vi "Generic command handler.vi"(8 "error in (no error)":errorcluster, 10 "Message in":refnum<class "GenericMessage.lvclass">, 11 "Tomo in":refnum<class "Tomo.lvclass">) -> (0 "error out":errorcluster, 2 "value":string, 3 "Tomo out":refnum<class "Tomo.lvclass">)   [LabVIEW 2012, in "Tomo.lvclass"]
doc: "The generic_command_handler processes the command 'generic'. Commands which are not part of the predefined list of commands fall under the 'generic' command for special activity."
uses:
  Tomo.lvclass
  <vilib>/Distrio/Murmex/GenericMessage/GenericMessage.lvclass
  <vilib>/Distrio/Murmex/Murmex/Murmex.lvclass
  Tomo.lvclass/Tomo.ctl
  <vilib>/Distrio/Murmex/StartMessage/StartMessage.lvclass
  Current activity.ctl
  file type.ctl
  notice type.ctl
  <vilib>/Distrio/Murmex/StopMessage/StopMessage.lvclass
  <vilib>/Distrio/Murmex/Message/Add or replace parameter.vi
  <vilib>/Distrio/Murmex/Message/Message.lvclass
  <vilib>/vision/NI_Vision_Development_Module.lvlib
panel:
  out "Image 2":T1(plugin-control)
  out "Image":T1(plugin-control)
  # "This method is called when the GENERIC\ntrigger is sent. \n\nOverride this method when your component needs to\nrespond to this trigger. \n\nCall parent for proper implementation"
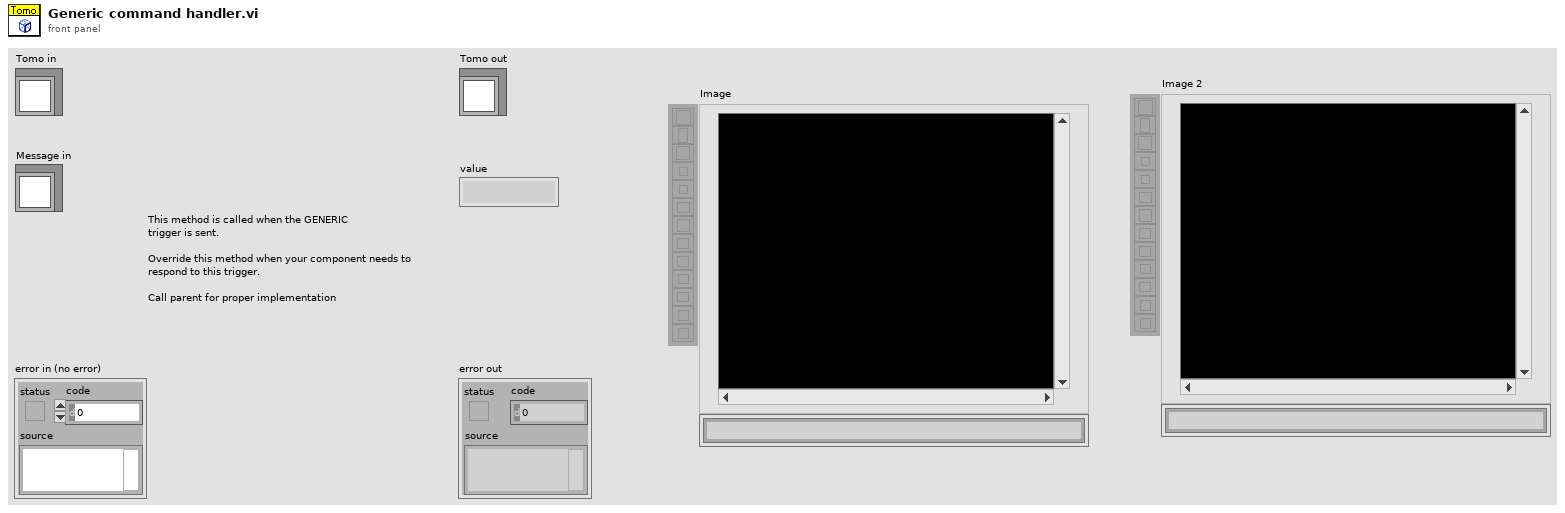
[diagram p1: front panel]
types:
  T1 = typedef "IMAQ Image.ctl" = refnum<image>
  T2 = typedef "Tomo.lvclass/Current activity.ctl" = enum16{"Idle", "Inter-stack motion", "Pre-tomo calculation", "Stack acquisition", "Stack preparation", "Pre-tomo stack acq", "Pre-tomo inter-stack"}
  T3 = typedef "Tomo.lvclass/file type.ctl" = enum16{"Volume map", "Completed stacks"}
  T4 = typedef "Tomo.lvclass/notice type.ctl" = enum16{"Tomography stopped", "Tomography error", "Tomography finished", "Timing issue", "Critical timing issue"}
  T5 = typedef "Tomo.lvclass/volume map.ctl" = enum16{"Cubic volume", "Custom volume", "Self-generate volume"}
  T6 = cluster{"Mean Value":sgl, "Standard Variation":sgl, "Minimal Value":sgl, "Maximal Value":sgl, "Area (calibrated)":sgl, "Area (pixels)":u32, "%":sgl, "Calibration Valid":bool}
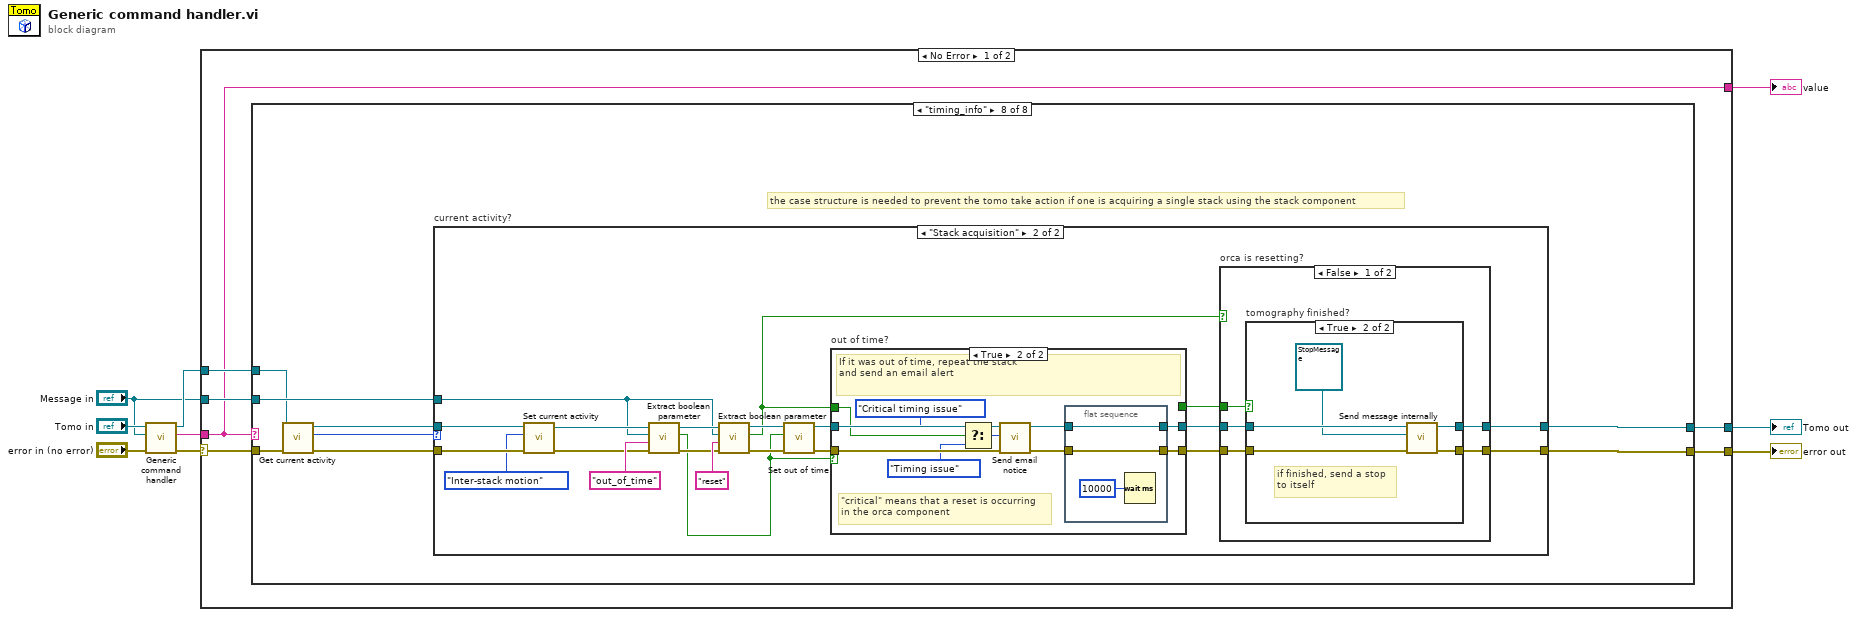
[diagram p0: block diagram]
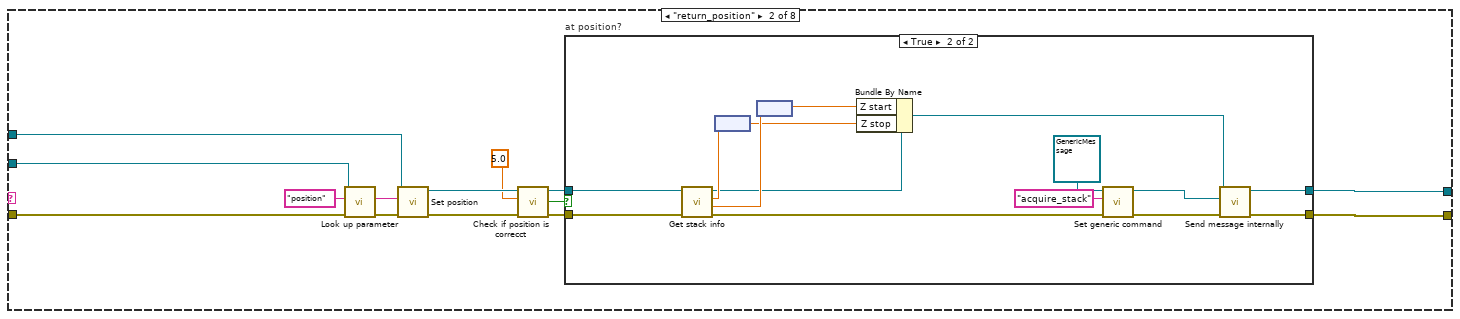
[diagram p3: hidden frame]
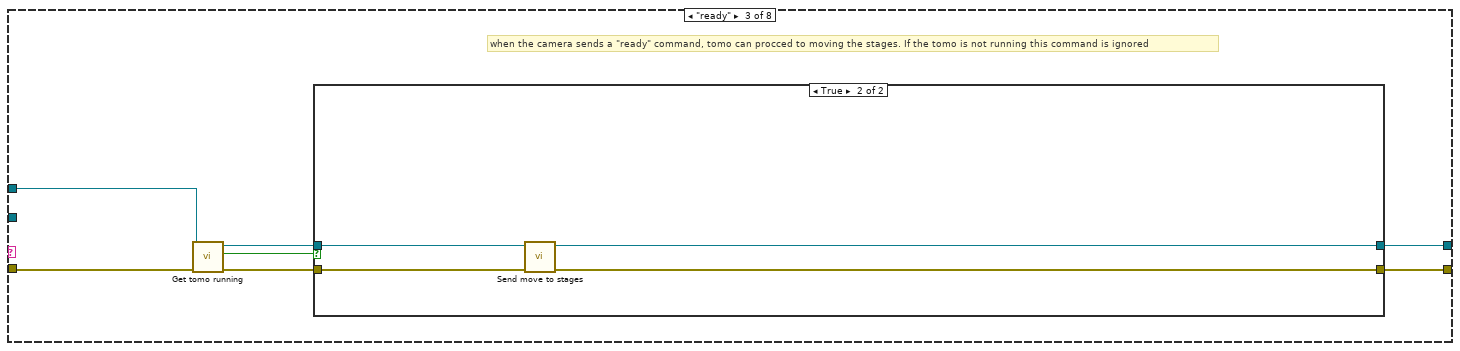
[diagram p5: hidden frame]
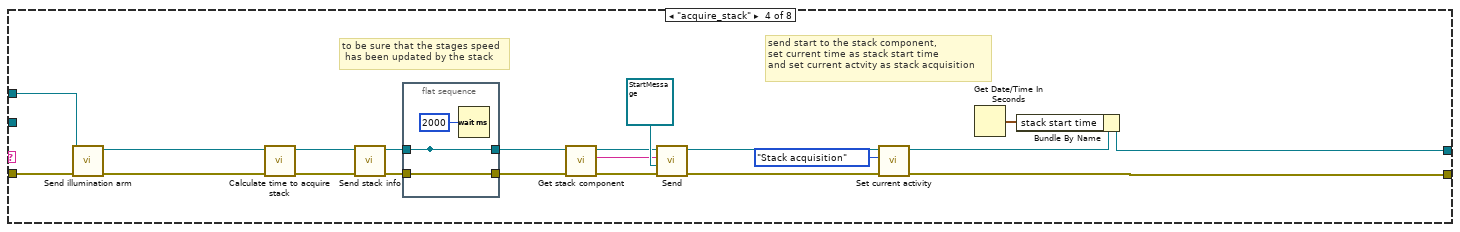
[diagram p7: hidden frame]
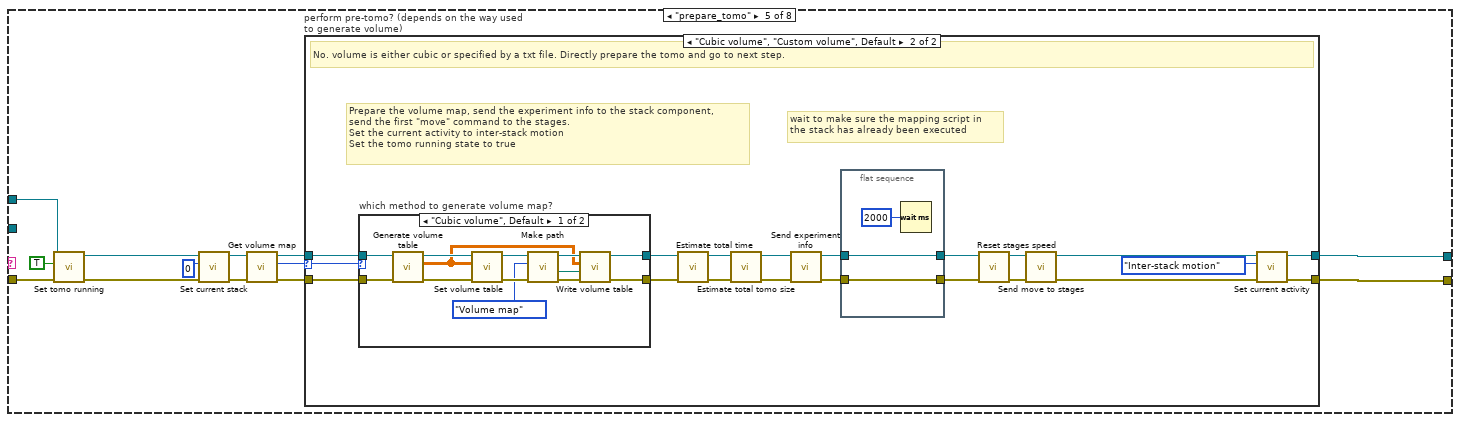
[diagram p8: hidden frame]
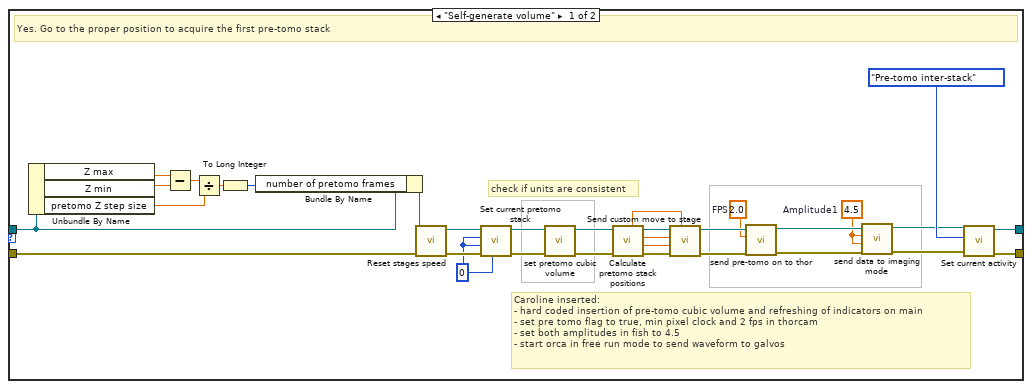
[diagram p9: hidden frame]
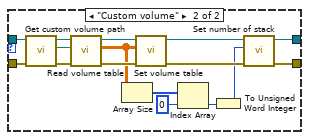
[diagram p10: hidden frame]
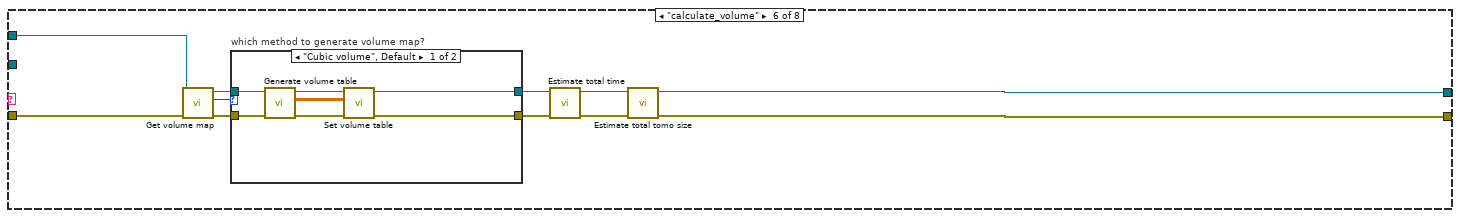
[diagram p11: hidden frame]
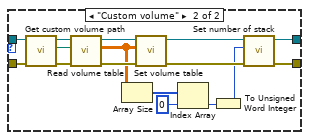
[diagram p12: hidden frame]
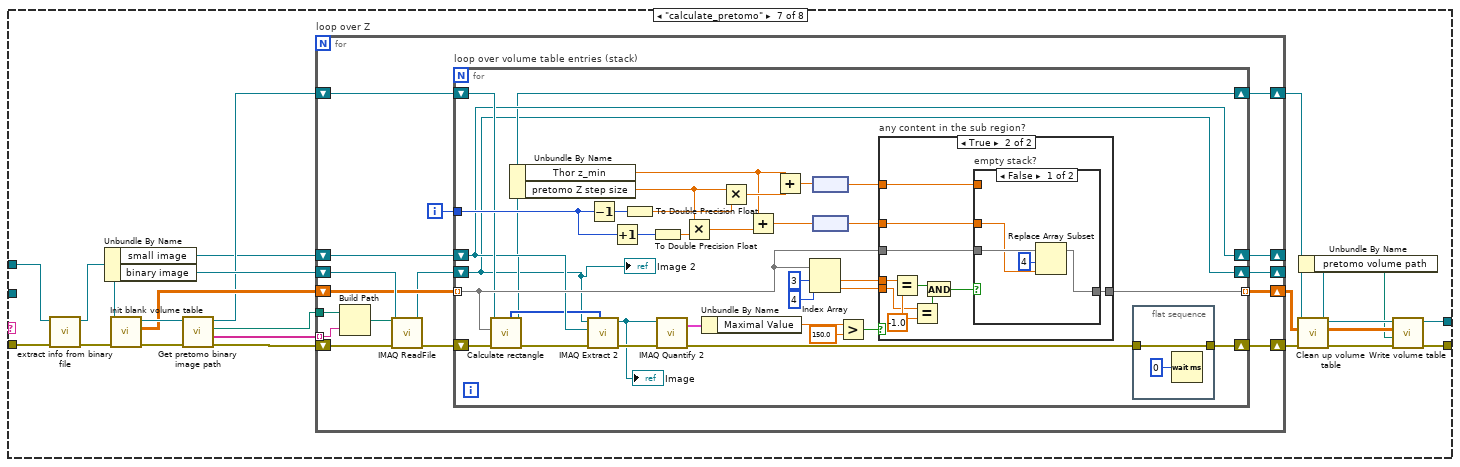
[diagram p13: hidden frame]
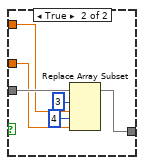
[diagram p15: hidden frame]
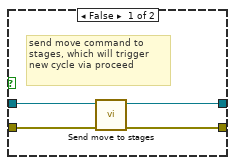
[diagram p17: hidden frame]
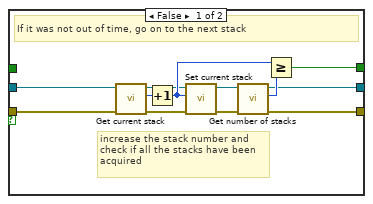
[diagram p19: hidden frame]
diagram:
  n1 = call-parent "Generic command handler.vi"("error in (no error)"="error in (no error)", "Message in"="Message in", "Murmex in"="Tomo in") -> ("error out"=w7:errorcluster, "value"=w6:string, "Murmex out"=w5:refnum<class "Tomo.lvclass">)  [unwired: 6 in]
  n2 = case shown="No Error" w7 {
    selector: w7 -> [w15 w384]
    tunnel: w6 -> [w11 w386]
    tunnel: w5 -> [w14 w385]
    tunnel: "Message in" -> [w13 _]
    tunnel: [w12 w385] -> w3
    tunnel: [w11 w386] -> w2
    tunnel: [w10 w384] -> w1
    frame No Error {
      n3 = case shown="\"timing_info\"" w11 {
        tunnel: w15 -> [w17 w31 w55 w66 w89 w186 w223 w316]
        tunnel: w14 -> [w16 w30 w54 w68 w90 w185 w221 w314]
        tunnel: w13 -> [_ w29 _ _ _ _ _ w319]
        tunnel: [w17 w19 w51 w79 w88 w183 w227 w317] -> w10
        tunnel: [w16 w18 w49 w62 w87 w184 w229 w318] -> w12
        frame Default {
        }
        frame "return_position" {
          n4 = call <vilib>:"Look up parameter.vi"("error in (no error)"=w31, "name"="position", "Message in"=w29) -> ("error out"=w27:errorcluster, "key"=w26:string)  [unwired: 5 in, 2 out]
          n5 = call-dynamic "Set position.vi"("error in (no error)"=w27, "XML in"=w26, "Tomo in"=w30) -> ("error out"=w25:errorcluster, "Tomo out"=w24:refnum<class "Tomo.lvclass">)  [unwired: 7 in]
          n6 = call-dynamic "Check if position is correcct.vi"("error in (no error)"=w25, "Tolerance (um)"=5.0 ("Tolerance"), "Tomo in"=w24) -> ("error out"=w21:errorcluster, "correct?"=w22:bool, "Tomo out"=w20:refnum<class "Tomo.lvclass">)  [unwired: 6 in]
          n7 = case "at position?" shown="True" w22 {
            tunnel: w21 -> [w33 w34]
            tunnel: w20 -> [w32 w35]
            tunnel: [w33 w48] -> w19
            tunnel: [w32 w47] -> w18
            frame False {
            }
            frame True {
              n8 = call-dynamic "Get stack info.vi"("error in (no error)"=w34, "Tomo in"=w35) -> ("error out"=w38:errorcluster, "Z start"=w45:dbl, "Z stop"=w46:dbl, "Tomo out"=w36:refnum<class "Tomo.lvclass">)  [unwired: 4 in, 2 out]
              n9 = node(w46) -> (w43:dbl[unit])
              n10 = node(w45) -> (w44:dbl[unit])
              n11 = Bundle By Name(cluster=w36, "Z start"=w44, "Z stop"=w43) -> (w37:refnum<class "Tomo.lvclass">)
              n12 = call <vilib>:"Set generic command.vi"("error in (no error)"=w38, "generic command"="acquire_stack", "GenericMessage in"=refnum<class "GenericMessage.lvclass"> refnum ("Distrio Murmex 1.2:GenericMessage")) -> ("error out"=w42:errorcluster, "GenericMessage out"=w39:refnum<class "GenericMessage.lvclass">)  [unwired: 7 in]
              n13 = call <vilib>:"Send message internally.vi"("error in (no error)"=w42, "Message"=w39, "Murmex in"=w37) -> ("error out"=w48:errorcluster, "Murmex out"=w47:refnum<class "Tomo.lvclass">)  [unwired: 7 in]
            }
          }
        }
        frame "ready" {
          # "when the camera sends a \"ready\" command, tomo can procced to moving the stages. If the tomo is not running this command is ignored"
          n14 = call-dynamic "Get tomo running.vi"("error in (no error)"=w55, "Tomo in"=w54) -> ("error out"=w52:errorcluster, "tomo running?"=w53:bool, "Tomo out"=w50:refnum<class "Tomo.lvclass">)  [unwired: 7 in]
          n15 = case shown="True" w53 {
            tunnel: w52 -> [w56 w61]
            tunnel: [w56 w60] -> w51
            tunnel: w50 -> [w57 w59]
            tunnel: [w57 w58] -> w49
            frame False {
            }
            frame True {
              n16 = call-dynamic "Send move to stages.vi"("error in (no error)"=w61, "Tomo in"=w59) -> ("error out"=w60:errorcluster, "Tomo out"=w58:refnum<class "Tomo.lvclass">)  [unwired: 8 in]
            }
          }
        }
        frame "acquire_stack" {
          # "to be sure that the stages speed\n has been updated by the stack"
          # "send start to the stack component,\nset current time as stack start time\nand set current actvity as stack acquisition"
          n17 = call-dynamic "Send illumination arm.vi"("error in (no error)"=w66, "Tomo in"=w68) -> ("error out"=w74:errorcluster, "Tomo out"=w73:refnum<class "Tomo.lvclass">)  [unwired: 8 in]
          n18 = call-dynamic "Calculate time to acquire stack.vi"("error in (no error)"=w74, "Tomo in"=w73) -> ("error out"=w65:errorcluster, "Tomo out"=w69:refnum<class "Tomo.lvclass">)  [unwired: 8 in]
          n19 = call-dynamic "Send stack info.vi"("error in (no error)"=w65, "Tomo in"=w69) -> ("error out"=w72:errorcluster, "Tomo out"=w71:refnum<class "Tomo.lvclass">)  [unwired: 8 in]
          n20 = flat-sequence {
            tunnel: [w85] -> w64
            tunnel: w72 -> [w85]
            tunnel: w71 -> [w83]
            tunnel: [w83] -> _
            tunnel: [w83] -> w67
            frame #0 {
              n21 = Wait (ms)(milliseconds to wait=u32 2000) -> ()  [unwired: 1 out]
            }
          }
          n22 = call-dynamic "Get stack component.vi"("error in (no error)"=w64, "Tomo in"=w67) -> ("error out"=w75:errorcluster, "stack component"=w81:string, "Tomo out"=w76:refnum<class "Tomo.lvclass">)  [unwired: 7 in]
          n23 = call <vilib>:"Send.vi"("error in (no error)"=w75, "Message"=refnum<class "StartMessage.lvclass"> refnum ("Message in"), "recipient"=w81, "Murmex in"=w76) -> ("error out"=w80:errorcluster, "Murmex out"=w78:refnum<class "Tomo.lvclass">)  [unwired: 6 in]
          n24 = call-dynamic "Set current activity.vi"("error in (no error)"=w80, "Current activity"=Current_activity."Stack acquisition", "Tomo in"=w78) -> ("error out"=w79:errorcluster, "Tomo out"=w63:refnum<class "Tomo.lvclass">)  [unwired: 7 in]
          n25 = Get Date/Time In Seconds() -> (seconds since 1Jan1904=w70:timestamp)
          n26 = Bundle By Name(cluster=w63, "stack start time"=w70) -> (w62:refnum<class "Tomo.lvclass">)
        }
        frame "prepare_tomo" {
          n27 = call-dynamic "Set tomo running.vi"("error in (no error)"=w89, "tomo running?"=TRUE, "Tomo in"=w90) -> ("error out"=w91:errorcluster, "Tomo out"=w92:refnum<class "Tomo.lvclass">)  [unwired: 7 in]
          n28 = call-dynamic "Set current stack.vi"("error in (no error)"=w91, "Current stack"=u16 0, "Tomo in"=w92) -> ("error out"=w95:errorcluster, "Tomo out"=w96:refnum<class "Tomo.lvclass">)  [unwired: 7 in]
          n29 = call-dynamic "Get volume map.vi"("error in (no error)"=w95, "Tomo in"=w96) -> ("error out"=w98:errorcluster, "Volume map"=w86:T5, "Tomo out"=w97:refnum<class "Tomo.lvclass">)  [unwired: 7 in]
          n30 = case "perform pre-tomo? (depends on the way used to generate volume)" shown="\"Cubic volume\", \"Custom volume\", Default" w86 {
            selector: w86 -> [_ w131]
            tunnel: w98 -> [w111 w150]
            tunnel: w97 -> [w112 w149]
            tunnel: [w123 w141] -> w88
            tunnel: [w122 w139] -> w87
            frame "Self-generate volume" {
              w105 = 2.0  # FPS
              w106 = 4.5  # Amplitude1
              w113 = 0 ("current x stack")
              # "Caroline inserted:\n- hard coded insertion of pre-tomo cubic volume and refreshing of indicators on main\n- set pre tomo flag to true, min pixel clock and 2 fps in thorcam\n- set both amplitudes in fish to 4.5\n- start orca in free run mode to send waveform to galvos"
              # "check if units are consistent"
              # "Yes. Go to the proper position to acquire the first pre-tomo stack"
              n31 = Unbundle By Name(w112) -> ("Z max"=w120:dbl[unit], "Z min"=w119:dbl[unit], "pretomo Z step size"=w117:dbl[unit])
              n32 = Subtract(x=w120, y=w119) -> (x-y=w118:dbl[unit])
              n33 = Divide(x=w118, y=w117) -> (x/y=w114:dbl)
              n34 = To Long Integer(number=w114) -> (32bit integer=w115:i32)
              n35 = Bundle By Name(cluster=w112, "number of pretomo frames"=w115) -> (w116:refnum<class "Tomo.lvclass">)
              n36 = call-dynamic "Reset stages speed.vi"("error in (no error)"=w111, "Tomo in"=w116) -> ("error out"=w130:errorcluster, "Tomo out"=w129:refnum<class "Tomo.lvclass">)  [unwired: 8 in]
              n37 = call-dynamic "Set current pretomo stack.vi"("z step number"=w113, "error in (no error)"=w130, "current y stack"=w113, "current x stack"=w113, "Tomo in"=w129) -> ("error out"=w102:errorcluster, "Tomo out"=w104:refnum<class "Tomo.lvclass">)  [unwired: 5 in]
              n38 = call-dynamic "set pretomo cubic volume.vi"("error in (no error)"=w102, "Tomo in"=w104) -> ("error out"=w101:errorcluster, "Tomo out"=w103:refnum<class "Tomo.lvclass">)  [unwired: 8 in]
              n39 = call-dynamic "Calculate pretomo stack positions.vi"("error in (no error)"=w101, "Tomo in"=w103) -> ("error out"=w127:errorcluster, "Y pos"=w124:dbl[unit], "X pos"=w125:dbl[unit], "Tomo out"=w128:refnum<class "Tomo.lvclass">, "Z pos"=w126:dbl[unit])  [unwired: 5 in]
              n40 = call-dynamic "Send custom move to stage.vi"("Z pos"=w126, "error in (no error)"=w127, "Y pos"=w124, "X pos"=w125, "Tomo in"=w128) -> ("error out"=w110:errorcluster, "Tomo out"=w109:refnum<class "Tomo.lvclass">)  [unwired: 5 in]
              n41 = call-dynamic "send pre-tomo on to thor.vi"("error in (no error)"=w110, "FPS"=w105, "Tomo in"=w109) -> ("error out"=w107:errorcluster, "Tomo out"=w108:refnum<class "Tomo.lvclass">)  [unwired: 7 in]
              n42 = call-dynamic "send data to imaging mode.vi"("error in (no error)"=w107, "Amplitude2"=w106, "Amplitude1"=w106, "Tomo in"=w108) -> ("error out"=w100:errorcluster, "Tomo out"=w99:refnum<class "Tomo.lvclass">)  [unwired: 6 in]
              n43 = call-dynamic "Set current activity.vi"("error in (no error)"=w100, "Current activity"=Current_activity."Pre-tomo inter-stack", "Tomo in"=w99) -> ("error out"=w123:errorcluster, "Tomo out"=w122:refnum<class "Tomo.lvclass">)  [unwired: 7 in]
            }
            frame "Cubic volume", "Custom volume", Default {
              # "wait to make sure the mapping script in \nthe stack has already been executed"
              # "Prepare the volume map, send the experiment info to the stack component,\nsend the first \"move\" command to the stages.\nSet the current activity to inter-stack motion\nSet the tomo running state to true"
              # "No. volume is either cubic or specified by a txt file. Directly prepare the tomo and go to next step."
              n44 = case "which method to generate volume map?" shown="\"Cubic volume\", Default" w131 {
                tunnel: w150 -> [w165 w180]
                tunnel: w149 -> [w166 w178]
                tunnel: [w155 w172] -> w147
                tunnel: [w154 w174] -> w148
                frame "Cubic volume", Default {
                  n45 = call-dynamic "Generate volume table.vi"("error in (no error)"=w165, "Tomo in"=w166) -> ("error out"=w163:errorcluster, "Volume table"=w156:dbl[][], "Tomo out"=w164:refnum<class "Tomo.lvclass">)  [unwired: 7 in]
                  n46 = call-dynamic "Set volume table.vi"("error in (no error)"=w163, "Volume map in"=w156, "Tomo in"=w164) -> ("error out"=w161:errorcluster, "Tomo out"=w162:refnum<class "Tomo.lvclass">)  [unwired: 7 in]
                  n47 = call-dynamic "Make path.vi"("error in (no error)"=w161, "File type"=file_type."Volume map", "Tomo in"=w162) -> ("error out"=w158:errorcluster, "path"=w157:path, "Tomo out"=w159:refnum<class "Tomo.lvclass">)  [unwired: 6 in]
                  n48 = call-dynamic "Write volume table.vi"("error in (no error)"=w158, "File name"=w157, "Volume map"=w156, "Tomo in"=w159) -> ("error out"=w154:errorcluster, "Tomo out"=w155:refnum<class "Tomo.lvclass">)  [unwired: 6 in]
                }
                frame "Custom volume" {
                  n49 = call-dynamic "Get custom volume path.vi"("error in (no error)"=w180, "Tomo in"=w178) -> ("error out"=w179:errorcluster, "Custom volume path"=w176:path, "Tomo out"=w177:refnum<class "Tomo.lvclass">)  [unwired: 7 in]
                  n50 = call "Read volume table.vi"("error in (no error)"=w179, "File path"=w176, "Tomo in"=w177) -> ("error out"=w181:errorcluster, "System Array"=w168:dbl[][], "Tomo out"=w182:refnum<class "Tomo.lvclass">)  [unwired: 6 in]
                  n51 = Array Size(array=w168) -> (size(s)=w171:i32[])
                  n52 = call-dynamic "Set volume table.vi"("error in (no error)"=w181, "Volume map in"=w168, "Tomo in"=w182) -> ("error out"=w175:errorcluster, "Tomo out"=w173:refnum<class "Tomo.lvclass">)  [unwired: 7 in]
                  n53 = Index Array(array=w171, index=0) -> (element=w169:i32)
                  n54 = To Unsigned Word Integer(number=w169) -> (unsigned 16bit integer=w167:u16)
                  n55 = call-dynamic "Set number of stack.vi"("error in (no error)"=w175, "Number of stacks"=w167, "Tomo in"=w173) -> ("error out"=w174:errorcluster, "Tomo out"=w172:refnum<class "Tomo.lvclass">)  [unwired: 7 in]
                }
              }
              n56 = call-dynamic "Estimate total time.vi"("error in (no error)"=w148, "Tomo in"=w147) -> ("error out"=w135:errorcluster, "Tomo out"=w137:refnum<class "Tomo.lvclass">)  [unwired: 7 in, 1 out]
              n57 = call "Estimate total tomo size.vi"("error in (no error)"=w135, "Tomo in"=w137) -> ("error out"=w134:errorcluster, "Tomo out"=w136:refnum<class "Tomo.lvclass">)  [unwired: 7 in, 1 out]
              n58 = call-dynamic "Send experiment info.vi"("error in (no error)"=w134, "Tomo in"=w136) -> ("error out"=w142:errorcluster, "Tomo out"=w144:refnum<class "Tomo.lvclass">)  [unwired: 8 in]
              n59 = flat-sequence {
                tunnel: [w153] -> w145
                tunnel: w144 -> [w153]
                tunnel: [w152] -> w143
                tunnel: w142 -> [w152]
                frame #0 {
                  n60 = Wait (ms)(milliseconds to wait=u32 2000) -> ()  [unwired: 1 out]
                }
              }
              n61 = call-dynamic "Reset stages speed.vi"("error in (no error)"=w143, "Tomo in"=w145) -> ("error out"=w133:errorcluster, "Tomo out"=w132:refnum<class "Tomo.lvclass">)  [unwired: 8 in]
              n62 = call-dynamic "Send move to stages.vi"("error in (no error)"=w133, "Tomo in"=w132) -> ("error out"=w146:errorcluster, "Tomo out"=w140:refnum<class "Tomo.lvclass">)  [unwired: 8 in]
              n63 = call-dynamic "Set current activity.vi"("error in (no error)"=w146, "Current activity"=Current_activity."Inter-stack motion", "Tomo in"=w140) -> ("error out"=w141:errorcluster, "Tomo out"=w139:refnum<class "Tomo.lvclass">)  [unwired: 7 in]
            }
          }
        }
        frame "calculate_volume" {
          n64 = call-dynamic "Get volume map.vi"("error in (no error)"=w186, "Tomo in"=w185) -> ("error out"=w192:errorcluster, "Volume map"=w193:T5, "Tomo out"=w191:refnum<class "Tomo.lvclass">)  [unwired: 7 in]
          n65 = case "which method to generate volume map?" shown="\"Cubic volume\", Default" w193 {
            tunnel: w192 -> [w199 w214]
            tunnel: w191 -> [w200 w212]
            tunnel: [w195 w206] -> w189
            tunnel: [w194 w208] -> w190
            frame "Cubic volume", Default {
              n66 = call-dynamic "Generate volume table.vi"("error in (no error)"=w199, "Tomo in"=w200) -> ("error out"=w197:errorcluster, "Volume table"=w196:dbl[][], "Tomo out"=w198:refnum<class "Tomo.lvclass">)  [unwired: 7 in]
              n67 = call-dynamic "Set volume table.vi"("error in (no error)"=w197, "Volume map in"=w196, "Tomo in"=w198) -> ("error out"=w194:errorcluster, "Tomo out"=w195:refnum<class "Tomo.lvclass">)  [unwired: 7 in]
            }
            frame "Custom volume" {
              n68 = call-dynamic "Get custom volume path.vi"("error in (no error)"=w214, "Tomo in"=w212) -> ("error out"=w213:errorcluster, "Custom volume path"=w210:path, "Tomo out"=w211:refnum<class "Tomo.lvclass">)  [unwired: 7 in]
              n69 = call "Read volume table.vi"("error in (no error)"=w213, "File path"=w210, "Tomo in"=w211) -> ("error out"=w215:errorcluster, "System Array"=w202:dbl[][], "Tomo out"=w216:refnum<class "Tomo.lvclass">)  [unwired: 6 in]
              n70 = Array Size(array=w202) -> (size(s)=w205:i32[])
              n71 = call-dynamic "Set volume table.vi"("error in (no error)"=w215, "Volume map in"=w202, "Tomo in"=w216) -> ("error out"=w209:errorcluster, "Tomo out"=w207:refnum<class "Tomo.lvclass">)  [unwired: 7 in]
              n72 = Index Array(array=w205, index=0) -> (element=w203:i32)
              n73 = To Unsigned Word Integer(number=w203) -> (unsigned 16bit integer=w201:u16)
              n74 = call-dynamic "Set number of stack.vi"("error in (no error)"=w209, "Number of stacks"=w201, "Tomo in"=w207) -> ("error out"=w208:errorcluster, "Tomo out"=w206:refnum<class "Tomo.lvclass">)  [unwired: 7 in]
            }
          }
          n75 = call-dynamic "Estimate total time.vi"("error in (no error)"=w190, "Tomo in"=w189) -> ("error out"=w187:errorcluster, "Tomo out"=w188:refnum<class "Tomo.lvclass">)  [unwired: 7 in, 1 out]
          n76 = call "Estimate total tomo size.vi"("error in (no error)"=w187, "Tomo in"=w188) -> ("error out"=w183:errorcluster, "Tomo out"=w184:refnum<class "Tomo.lvclass">)  [unwired: 7 in, 1 out]
        }
        frame "calculate_pretomo" {
          n77 = call-dynamic "extract info from binary file.vi"("error in (no error)"=w223, "Tomo in"=w221) -> ("error out"=w222:errorcluster, "Tomo out"=w220:refnum<class "Tomo.lvclass">)  [unwired: 8 in]
          n78 = Unbundle By Name(w220) -> ("small image"=w233:T1, "binary image"=w236:T1)
          n79 = call-dynamic "Init blank volume table.vi"("error in (no error)"=w222, "Tomo in"=w220) -> ("error out"=w237:errorcluster, "blank volume table"=w235:dbl[][], "Tomo out"=w238:refnum<class "Tomo.lvclass">)  [unwired: 7 in]
          n80 = call-dynamic "Get pretomo binary image path.vi"("error in (no error)"=w237, "Tomo in"=w238) -> ("error out"=w219:errorcluster, "filenames"=w218:string[], "pretomo binary path"=w217:path, "Tomo out"=w234:refnum<class "Tomo.lvclass">)  [unwired: 6 in]
          n81 = for "loop over Z" {
            shift-right: [w243] -> w231
            shift-left: w219 -> [w254]
            shift-right: [w245] -> w230
            shift-left: w235 -> [w251]
            shift-right: [w244] -> w232
            shift-left: w234 -> [w249]
            shift-right: [w242] -> _
            shift-left: w233 -> [w247]
            shift-right: [w241] -> _
            shift-left: w236 -> [w253]
            tunnel: w218 -> [w240] mode=indexing
            tunnel: w217 -> [w239]
            i -> [w246]
            n82 = Build Path(base path=w239, name or relative path=w240) -> (appended path=w252:path)
            n83 = call "IMAQ ReadFile"("File Path"=w252, "error in (no error)"=w254, "Image"=w253) -> ("error out"=w250:errorcluster, "Image Out"=w248:T1)  [unwired: 4 in, 3 out]
            n84 = for "loop over volume table entries (stack)" {
              tunnel: w251 -> [w277] mode=indexing
              shift-right: [w258] -> w243
              shift-left: w250 -> [w288]
              tunnel: w246 -> [w272]
              tunnel: [w263] -> w245 mode=indexing
              shift-right: [w259] -> w244
              shift-left: w249 -> [w262]
              shift-right: [w261] -> w242
              shift-left: w247 -> [w261]
              shift-right: [w255] -> w241
              shift-left: w248 -> [w255]
              n85 = call-dynamic "Calculate rectangle.vi"("error in (no error)"=w288, "xyzs array"=w277, "Tomo in"=w262) -> ("error out"=w287:errorcluster, "Tomo out"=w259:refnum<class "Tomo.lvclass">, "rectangle"=w260:i32[])  [unwired: 6 in]
              n86 = Unbundle By Name(w259) -> ("Thor z_min"=w265:dbl[unit], "pretomo Z step size"=w269:dbl[unit])
              n87 = call "IMAQ Extract 2"("Optional Rectangle"=w260, "error in (no error)"=w287, "Image Dst"=w261, "Image Src"=w255) -> ("error out"=w286:errorcluster, "Image Dst Out"=w256:T1)  [unwired: 6 in]
              "Image" <- w256
              n88 = Decrement(x=w272) -> (x-1=w275:i32)
              n89 = Increment(x=w272) -> (x+1=w271:i32)
              n90 = To Double Precision Float(number=w275) -> (double precision float=w276:dbl)
              n91 = To Double Precision Float(number=w271) -> (double precision float=w270:dbl)
              n92 = call "IMAQ Quantify 2"("error in (no error)"=w286, "Image"=w256) -> ("error out"=w257:errorcluster, "Global Report"=w285:T6)  [unwired: 7 in, 1 out]
              n93 = Multiply(x=w269, y=w270) -> (x*y=w267:dbl[unit])
              n94 = Unbundle By Name(w285) -> ("Maximal Value"=w282:sgl)
              n95 = Multiply(x=w269, y=w276) -> (x*y=w268:dbl[unit])
              n96 = Add(x=w265, y=w267) -> (x+y=w266:dbl[unit])
              n97 = Add(x=w265, y=w268) -> (x+y=w274:dbl[unit])
              n98 = Index Array(array=w277, index #1=3 ("index"), index #2=4 ("index")) -> (element #1=w279:dbl, element #2=w278:dbl)
              n99 = node(w274) -> (w273:dbl)
              n100 = node(w266) -> (w264:dbl)
              n101 = Greater?(x=w282, y=sgl 150.0) -> (0:w280:bool)
              n102 = case "any content in the sub region?" shown="True" w280 {
                tunnel: w279 -> [_ w301]
                tunnel: w278 -> [_ w299]
                tunnel: w277 -> [w291 w298]
                tunnel: w273 -> [_ w297]
                tunnel: w264 -> [_ w295]
                tunnel: [w291 w296] -> w263
                frame False {
                }
                frame True {
                  w300 = -1.0 ("y")
                  n103 = Equal?(x=w301, y=w300) -> (x = y?=w293:bool)
                  n104 = Equal?(x=w299, y=w300) -> (x = y?=w294:bool)
                  n105 = And(x=w293, y=w294) -> (x .and. y?=w292:bool)
                  n106 = case "empty stack?" shown="False" w292 {
                    tunnel: w298 -> [w304 w311]
                    tunnel: w297 -> [_ w309]
                    tunnel: [w302 w308] -> w296
                    tunnel: w295 -> [w303 w306]
                    frame False {
                      n107 = Replace Array Subset(array=w304, new element=w303, index=4) -> (w302:dbl[])
                    }
                    frame True {
                      n108 = Replace Array Subset(array=w311, new element #1=w309, index #1=3 ("index"), new element #2=w306, index #2=4 ("index")) -> (w308:dbl[])
                    }
                  }
                }
              }
              n109 = flat-sequence {
                tunnel: [w290] -> w258
                tunnel: w257 -> [w290]
                frame #0 {
                  n110 = Wait (ms)(milliseconds to wait=u32 0) -> ()  [unwired: 1 out]
                }
              }
              "Image 2" <- w255
            }
          }
          n111 = call-dynamic "Clean up volume table.vi"("error in (no error)"=w231, "Volume table in"=w230, "Tomo in"=w232) -> ("error out"=w228:errorcluster, "Volume table out"=w226:dbl[][], "Tomo out"=w225:refnum<class "Tomo.lvclass">)  [unwired: 6 in]
          n112 = Unbundle By Name(w225) -> ("pretomo volume path"=w224:path)
          n113 = call-dynamic "Write volume table.vi"("error in (no error)"=w228, "File name"=w224, "Volume map"=w226, "Tomo in"=w225) -> ("error out"=w227:errorcluster, "Tomo out"=w229:refnum<class "Tomo.lvclass">)  [unwired: 6 in]
        }
        frame "timing_info" {
          # "the case structure is needed to prevent the tomo take action if one is acquiring a single stack using the stack component"
          n114 = call-dynamic "Get current activity.vi"("error in (no error)"=w316, "Tomo in"=w314) -> ("error out"=w315:errorcluster, "Current activity"=w312:T2, "Tomo out"=w313:refnum<class "Tomo.lvclass">)  [unwired: 7 in]
          n115 = case "current activity?" shown="\"Stack acquisition\"" w312 {
            tunnel: w319 -> [_ w324]
            tunnel: [w321 w340] -> w318
            tunnel: [w320 w339] -> w317
            tunnel: w315 -> [w320 w335]
            tunnel: w313 -> [w321 w334]
            frame "Idle", Default {
            }
            frame "Stack acquisition" {
              n116 = call-dynamic "Set current activity.vi"("error in (no error)"=w335, "Current activity"=Current_activity."Inter-stack motion", "Tomo in"=w334) -> ("error out"=w322:errorcluster, "Tomo out"=w326:refnum<class "Tomo.lvclass">)  [unwired: 7 in]
              n117 = call-dynamic "Extract boolean parameter.vi"("error in (no error)"=w322, "parameter"="out_of_time" ("name"), "Message in"=w324, "Tomo in"=w326) -> ("error out"=w328:errorcluster, "parameter"=w327:bool, "Tomo out"=w325:refnum<class "Tomo.lvclass">)  [unwired: 5 in]
              n118 = call-dynamic "Extract boolean parameter.vi"("error in (no error)"=w328, "parameter"="reset" ("name"), "Message in"=w324, "Tomo in"=w325) -> ("error out"=w332:errorcluster, "parameter"=w330:bool, "Tomo out"=w331:refnum<class "Tomo.lvclass">)  [unwired: 5 in]
              n119 = call-dynamic "Set out of time.vi"("error in (no error)"=w332, "out of time?"=w327, "Tomo in"=w331) -> ("error out"=w337:errorcluster, "Tomo out"=w336:refnum<class "Tomo.lvclass">)  [unwired: 7 in]
              n120 = case "out of time?" shown="True" w327 {
                tunnel: w337 -> [w363 w379]
                tunnel: w336 -> [w362 w380]
                tunnel: [w361 w374] -> w342
                tunnel: [w360 w372] -> w341
                tunnel: [w359 _] -> w338
                tunnel: w330 -> [_ w376]
                frame False {
                  # "increase the stack number and\ncheck if all the stacks have been\nacquired"
                  # "If it was not out of time, go on to the next stack"
                  n121 = call-dynamic "Get current stack.vi"("error in (no error)"=w363, "Tomo in"=w362) -> ("error out"=w365:errorcluster, "Current stack"=w366:u16, "Tomo out"=w364:refnum<class "Tomo.lvclass">)  [unwired: 7 in]
                  n122 = Increment(x=w366) -> (x+1=w370:u16)
                  n123 = call-dynamic "Set current stack.vi"("error in (no error)"=w365, "Current stack"=w370, "Tomo in"=w364) -> ("error out"=w367:errorcluster, "Tomo out"=w368:refnum<class "Tomo.lvclass">)  [unwired: 7 in]
                  n124 = call-dynamic "Get number of stacks.vi"("error in (no error)"=w367, "Tomo in"=w368) -> ("error out"=w361:errorcluster, "Number of stacks"=w369:u16, "Tomo out"=w360:refnum<class "Tomo.lvclass">)  [unwired: 7 in]
                  n125 = Greater Or Equal?(x=w370, y=w369) -> (x >= y?=w359:bool)
                }
                frame True {
                  # "\"critical\" means that a reset is occurring\nin the orca component"
                  # "If it was out of time, repeat the stack\nand send an email alert"
                  n126 = Select(t=notice_type."Critical timing issue" ("Notice type"), s=w376, f=notice_type."Timing issue" ("Notice type")) -> (s? t:f=w375:T4)
                  n127 = call-dynamic "Send email notice.vi"("error in (no error)"=w379, "Notice type"=w375, "Tomo in"=w380) -> ("error out"=w373:errorcluster, "Tomo out"=w371:refnum<class "Tomo.lvclass">)  [unwired: 7 in]
                  n128 = flat-sequence {
                    tunnel: [w383] -> w374
                    tunnel: w373 -> [w383]
                    tunnel: [w382] -> w372
                    tunnel: w371 -> [w382]
                    frame #0 {
                      n129 = Wait (ms)(milliseconds to wait=u32 10000) -> ()  [unwired: 1 out]
                    }
                  }
                }
              }
              n130 = case "orca is resetting?" shown="False" w330 {
                tunnel: w342 -> [w347 w358]
                tunnel: w341 -> [w346 w357]
                tunnel: [w345 w357] -> w340
                tunnel: [w344 w358] -> w339
                tunnel: w338 -> [w343 _]
                frame False {
                  n131 = case "tomography finished?" shown="True" w343 {
                    tunnel: w347 -> [w351 w356]
                    tunnel: w346 -> [w350 w353]
                    tunnel: [w349 w354] -> w345
                    tunnel: [w348 w355] -> w344
                    frame False {
                      # "send move command to stages, which will trigger new cycle via proceed"
                      n132 = call-dynamic "Send move to stages.vi"("error in (no error)"=w351, "Tomo in"=w350) -> ("error out"=w348:errorcluster, "Tomo out"=w349:refnum<class "Tomo.lvclass">)  [unwired: 8 in]
                    }
                    frame True {
                      # "if finished, send a stop\nto itself"
                      n133 = call <vilib>:"Send message internally.vi"("error in (no error)"=w356, "Message"=refnum<class "StopMessage.lvclass"> refnum ("Message in"), "Murmex in"=w353) -> ("error out"=w355:errorcluster, "Murmex out"=w354:refnum<class "Tomo.lvclass">)  [unwired: 7 in]
                    }
                  }
                }
                frame True {
                  # "do nothing. Orca will tell\nyou when it's ready"
                }
              }
            }
          }
        }
      }
    }
    frame Error {
    }
  }
  "error out" <- w1
  "Tomo out" <- w3
  "value" <- w2
